vi "Sweep Control.vi"() -> ()   [LabVIEW 2019, in "SweepControl.lvclass"]
doc: "- Priority 0 is the fastest loop\n- You can put multiple scan names in one priority.\n- OFF has to be the last priority\n- Choose an Experiment (Lockin_Sweep, IV, etc) to run at each Scan Setting\n- Open the Exeriment subVIs to choose settings"
uses:
  SweepControl.lvclass
  Typedefs/Enum - Priority.ctl
  Typedefs/Enum - Action.ctl
  Typedefs/Cluster - ScanControl.ctl
  Typedefs/ScanControl.ctl
  Typedefs/Cluster - ScanParamters.ctl
  Typedefs/ScanParamters.ctl
  Typedefs/Enum - Experiments.ctl
  Typedefs/Sweep Control JSON--Cluster.ctl
  Control Experiment/Control Experiment.lvclass
  Typedefs/Enum - PostAction.ctl
  Typedefs/PostAction.ctl
  Typedefs/Enum - PostAction - 2.ctl
  Typedefs/Cluster - Sweep Control.ctl
panel:
  out "Repeat #":i32
  in  "Repeat Experiment":i32=100 caption="Repeat Experiment (at each parameter)" min=1
  in  "Stop":bool
  in  "Scan parameters 2":T1[](array[typedef]) {"Rate" format="%.2f"; "Step" format="%#_6p"; "End" format="%#_6p"; "Start" format="%#_6p"}
  in  "OK":bool
  in  "Experiment Description":string="T = 20 K\nRainbow 2 power = 250 uW before int\n50 second time delay scan [-0.5 ps, 0.5 ps]\n15 averages per Vgr value\n\ntop nanojunction Vsd = -0.7 V\nbottom nanojunction Vsd = -0.5 V\nVgr = 0 V\n\nSweep Vnw from 0 V to -1 V, -100 mV step\n\n"
  in  "Experiment subVI":T5=enum."THz_DelayLine"
  in  "Post action (indexing priority)":T6=[enum."Do Nothing", enum."Do Nothing", enum."Do Nothing", enum."Do Nothing"]
  in  "Experiment Folder (## - Description)":string="35 - sweep Vnw bottom 100 repeats "
  in  "Scan parameters":T8=[{"Start"=-0.5, "End"=-1.5, "Step"=0.1, "Rate"=0.0, "wait (ms/mK)"=2000, "Address"="Dev2/ao0", "channel"=5}, {"Start"=0.0, "End"=-1.0, "Step"=0.1, "Rate"=0.0, "wait (ms/mK)"=2000, "Address"="Dev2/ao0", "channel"=7}, {"Start"=0.2, "End"=0.3, "Step"=0.025, "Rate"=2.0, "wait (ms/mK)"=250, "Address"="Dev2/ao0", "channel"=3}, {"Start"=0.0, "End"=10000.0, "Step"=5000.0, "Rate"=0.0, "wait (ms/mK)"=0, "Address"="Dev2/ao0", "channel"=3}] {"Rate" format="%.2f"; "Step" format="%#_6p"; "End" format="%#_6p"; "Start" format="%#_6p"}
  in  "Scan control":T10=[{"Priority"=enum."Priority 0", "Scan name"=enum."Lockin Bias"}, {"Priority"=enum."Priority 0", "Scan name"=enum."Lockin Bias"}, {"Priority"=enum."Priority 2", "Scan name"=enum."OFF"}, {"Priority"=enum."Priority 3", "Scan name"=enum."OFF"}]
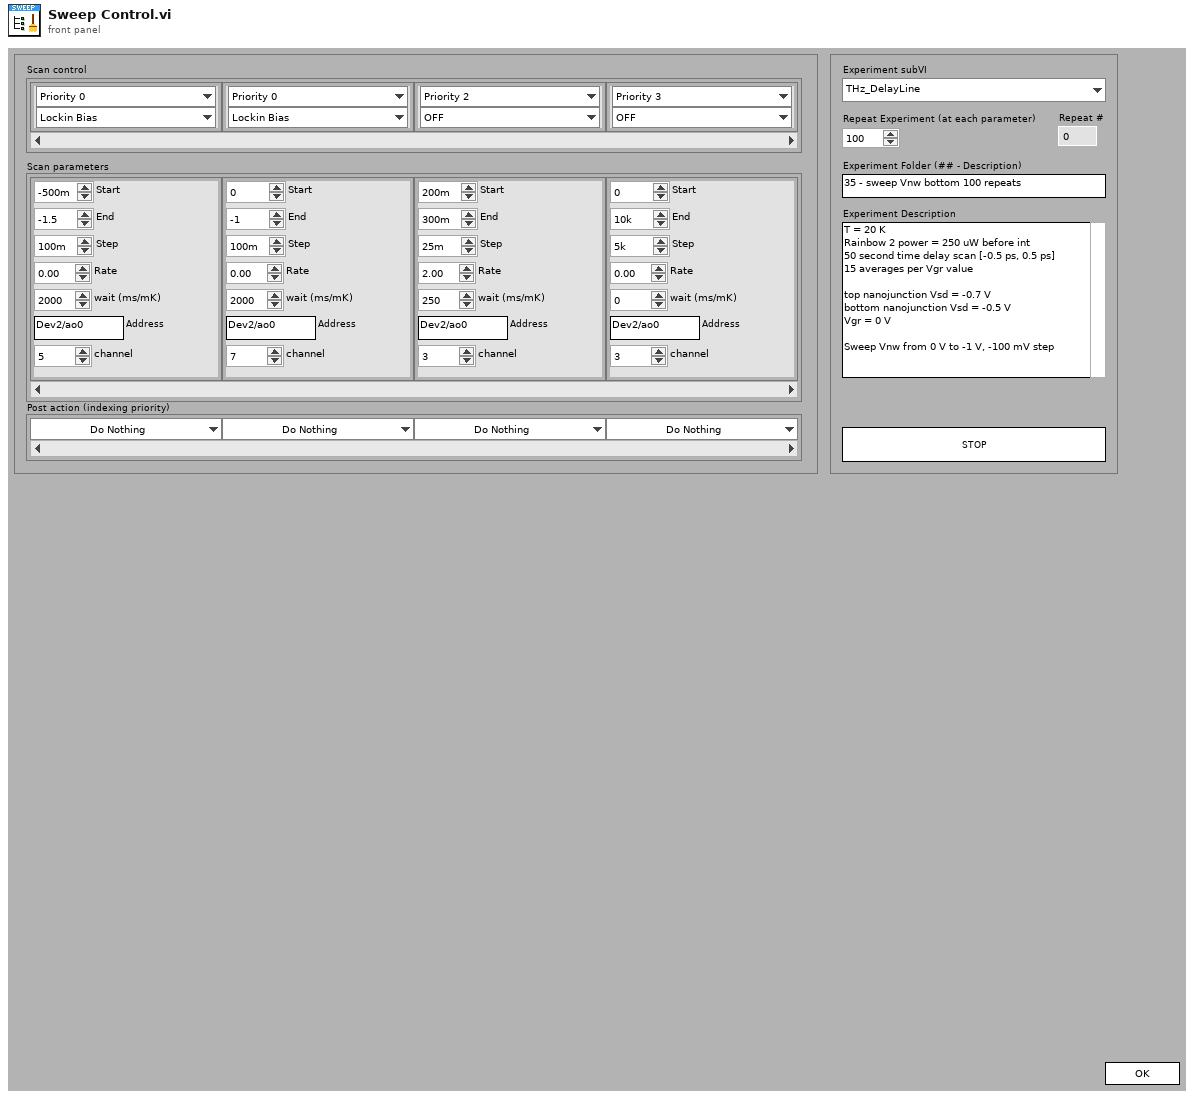
[diagram p1: front panel]
types:
  T1 = typedef "SweepControl.lvclass/Cluster - Sweep Control.ctl" = cluster{"Start":dbl, "End":dbl, "Step":dbl, "Rate":dbl, "wait (ms/mK)":u32, "Address":string, "Priority":T2, "Scan name":T3, "Post Actions":T4[], "channel":i32}
  T2 = typedef "SweepControl.lvclass/Enum - Priority.ctl" = enum16{"Priority 0", "Priority 1", "Priority 2", "Priority 3", "Priority 4", "Priority 5"}
  T3 = typedef "SweepControl.lvclass/Enum - Action.ctl" = enum16{"OFF", "time", "Lockin Amplitude", "Lockin Frequency", "Lockin Bias", "Delay", "Strain", "DAQ Bias", "Magnet Field", "Temperature", "MW f1", "MW f2", "MW Amplitude1", "MW Amplitude2"}
  T4 = typedef "SweepControl.lvclass/Enum - PostAction - 2.ctl" = enum16{"Do Nothing", "Wait (time)", "Wait (Temperature)", "Wait (<T ; B sweep)", "Wait (Magnet)"}
  T5 = typedef "SweepControl.lvclass/Enum - Experiments.ctl" = enum16{"IV", "IV_Fast", "IV_Sweep", "THz_DelayLine", "Lockin_Vsg", "Lockin_Sweep", "Lockin_Time", "AI WFM time", "Lockin (experimental)"}
  T6 = typedef "SweepControl.lvclass/PostAction.ctl" = T7[]
  T7 = typedef "SweepControl.lvclass/Enum - PostAction.ctl" = enum16{"Do Nothing", "Wait (time)", "Wait (Temperature)", "Wait (<T ; B sweep)", "Wait (Magnet)"}
  T8 = typedef "SweepControl.lvclass/ScanParamters.ctl" = T9[]
  T9 = typedef "SweepControl.lvclass/Cluster - ScanParamters.ctl" = cluster{"Start":dbl, "End":dbl, "Step":dbl, "Rate":dbl, "wait (ms/mK)":u32, "Address":string, "channel":i32}
  T10 = typedef "SweepControl.lvclass/ScanControl.ctl" = T11[]
  T11 = typedef "SweepControl.lvclass/Cluster - ScanControl.ctl" = cluster{"Priority":T2, "Scan name":T3}
  T12 = enum32{"Invalid", "Standard", "Closed", "Hidden", "Minimized", "Maximized"}
  T13 = enum32{"invalid app kind", "Development System", "Run Time System", "Student Edition", "Embedded LabVIEW", "Evaluation", "Custom"}
  T14 = cluster{"Core":cluster{"Current VI Reference":refnum<vi>, "Close Panel on Exit?":bool}, "SweepControl":refnum<class "SweepControl.lvclass">}
  T15 = cluster{"Current VI Reference":refnum<vi>, "Close Panel on Exit?":bool}
  T16 = typedef "SweepControl.lvclass/Sweep Control JSON--Cluster.ctl" = cluster{"Experiment":T5, "Repeat Experiment":i32, "Scan control":T10, "Scan parameters":T8}
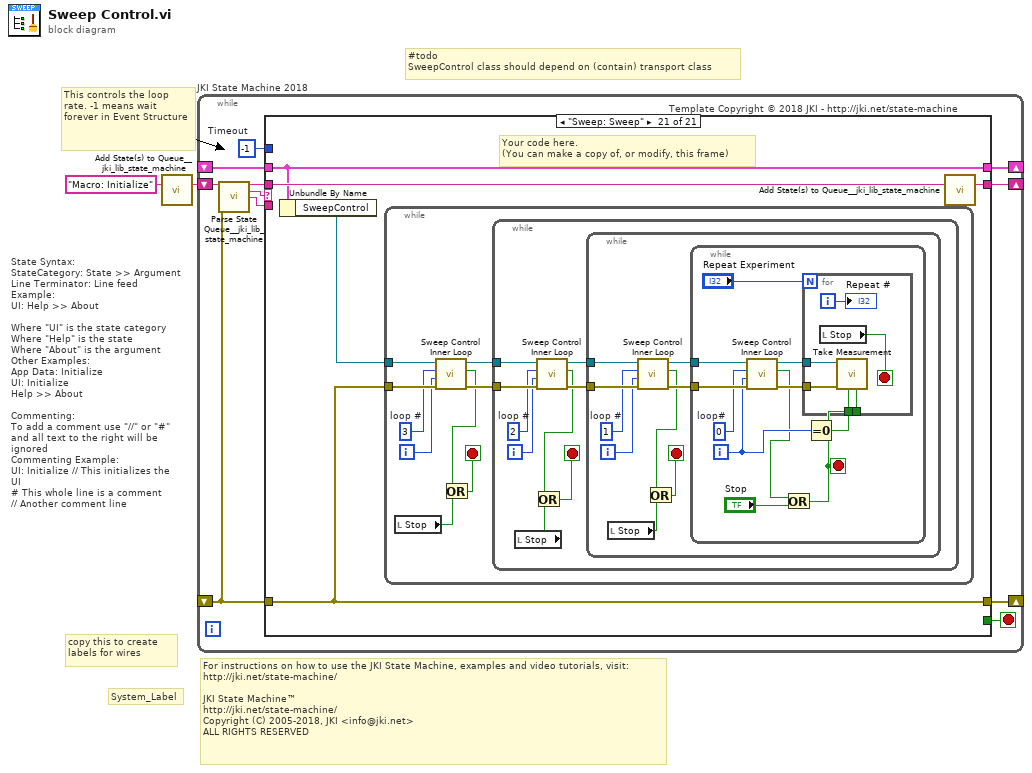
[diagram p0: block diagram]
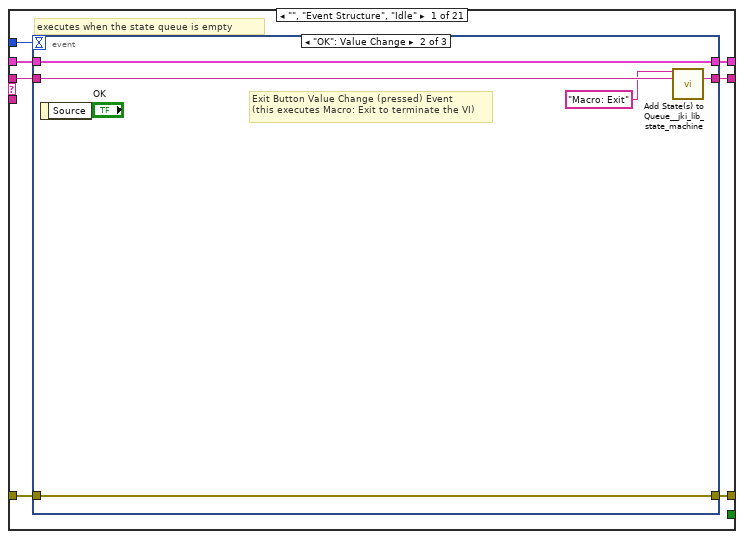
[diagram p2: hidden frame]
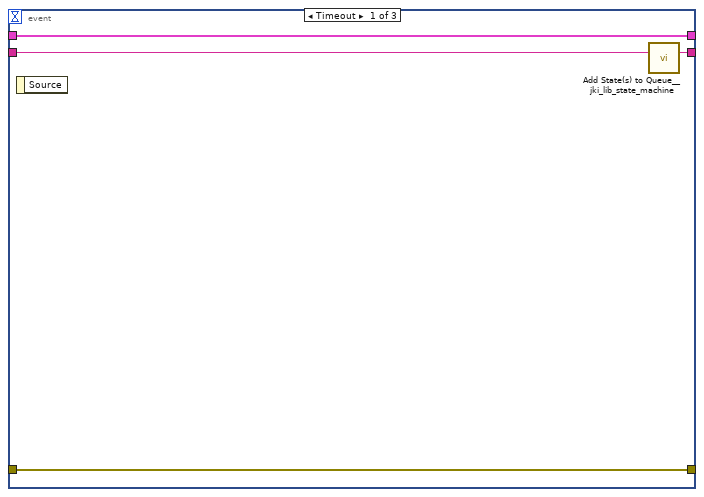
[diagram p3: hidden frame]
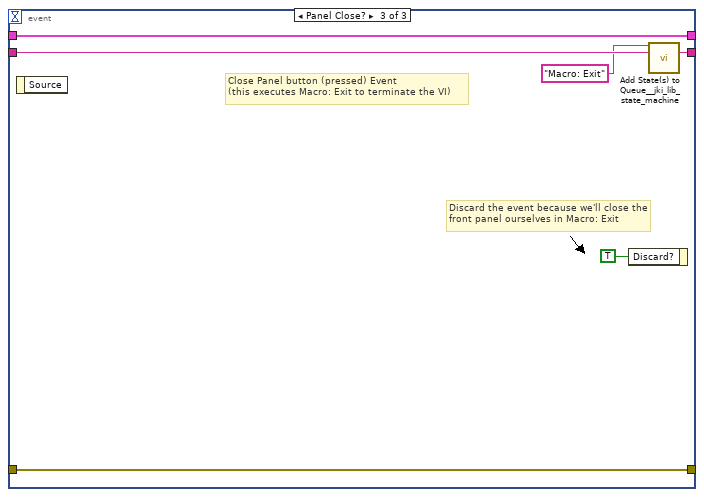
[diagram p4: hidden frame]
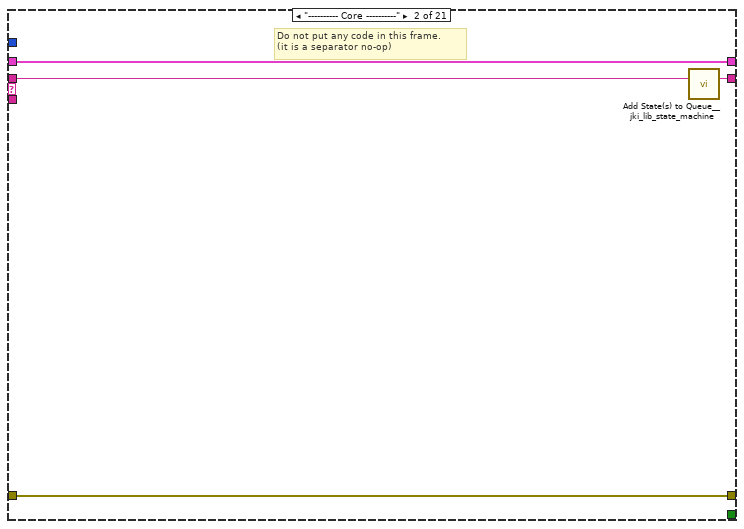
[diagram p5: hidden frame]
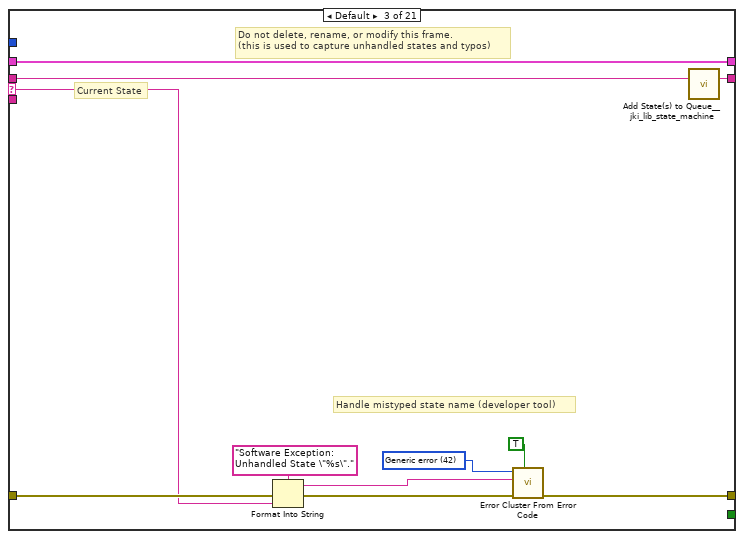
[diagram p6: hidden frame]
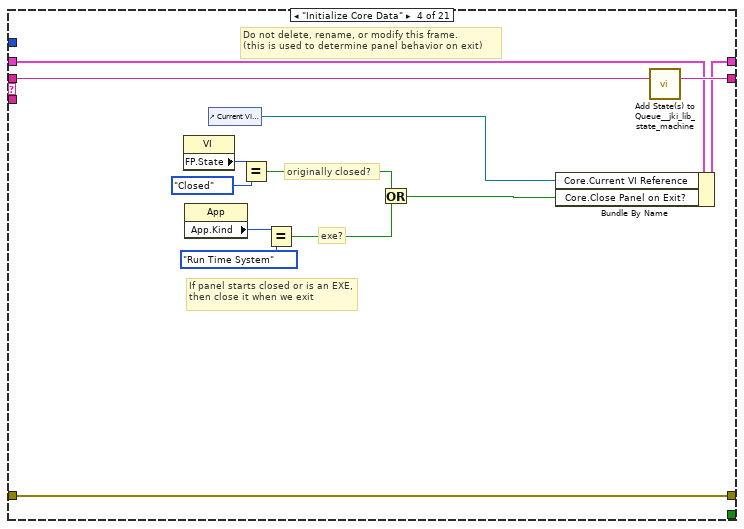
[diagram p7: hidden frame]
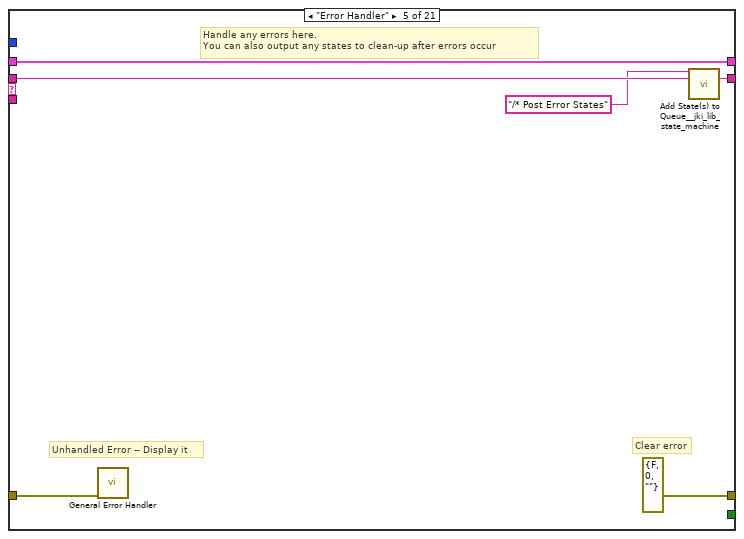
[diagram p8: hidden frame]
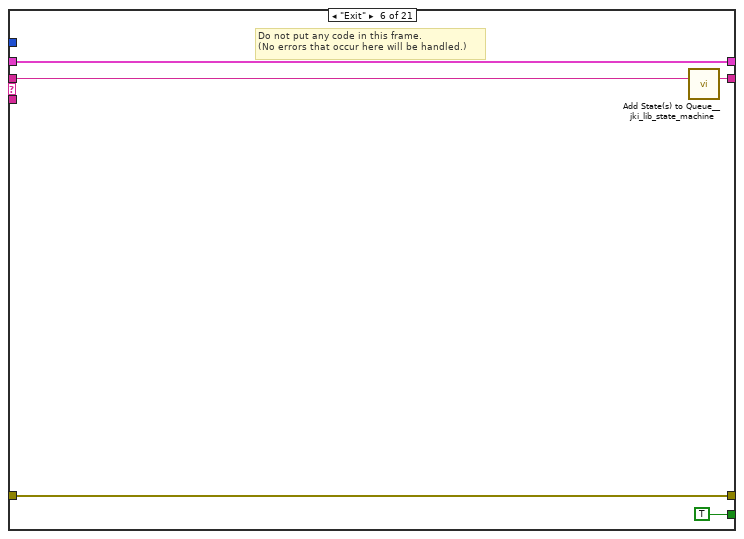
[diagram p9: hidden frame]
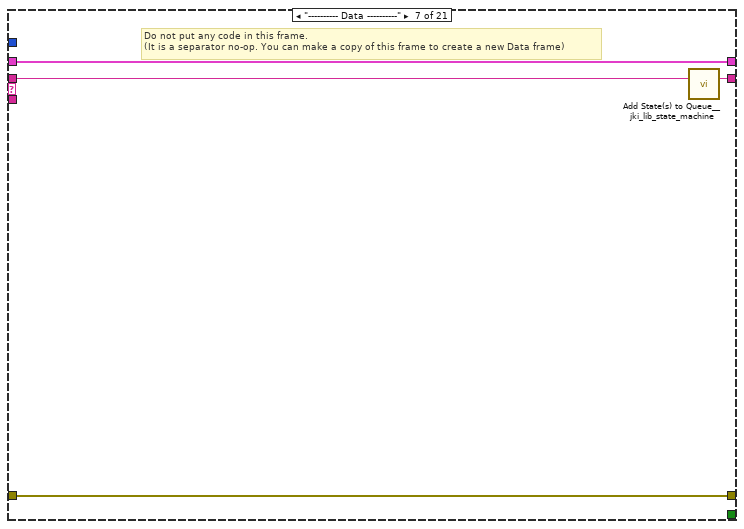
[diagram p10: hidden frame]
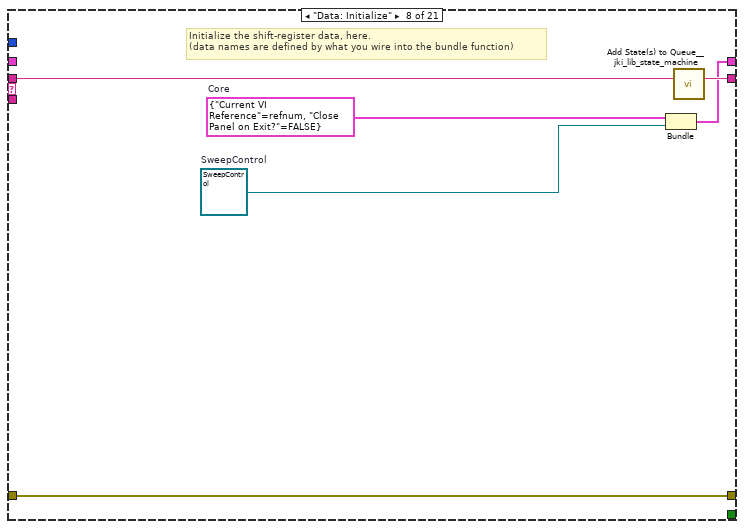
[diagram p11: hidden frame]
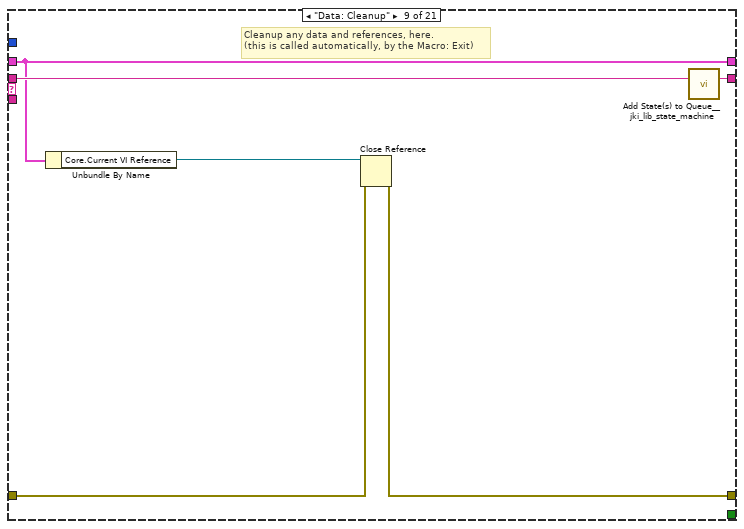
[diagram p12: hidden frame]
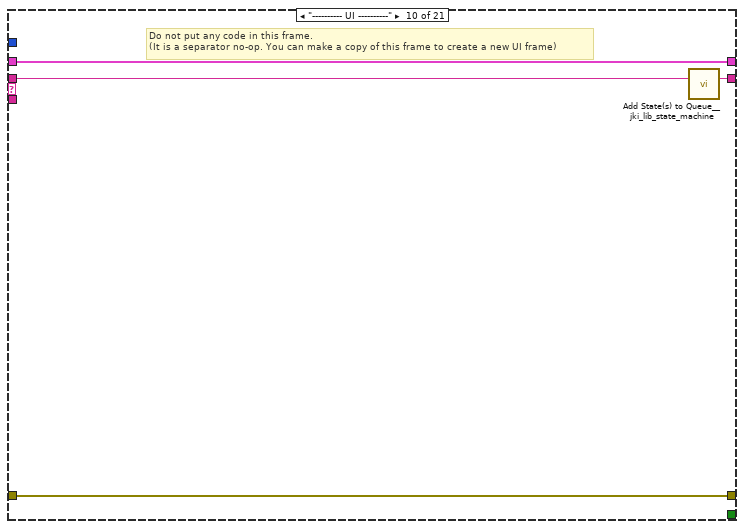
[diagram p13: hidden frame]
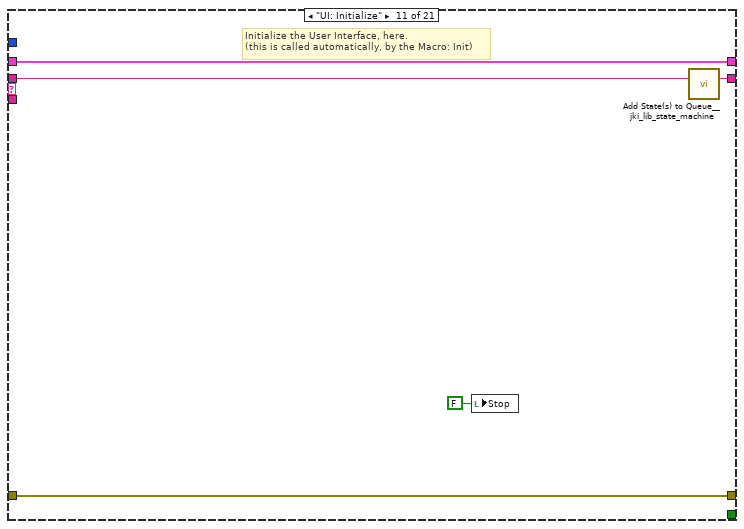
[diagram p14: hidden frame]
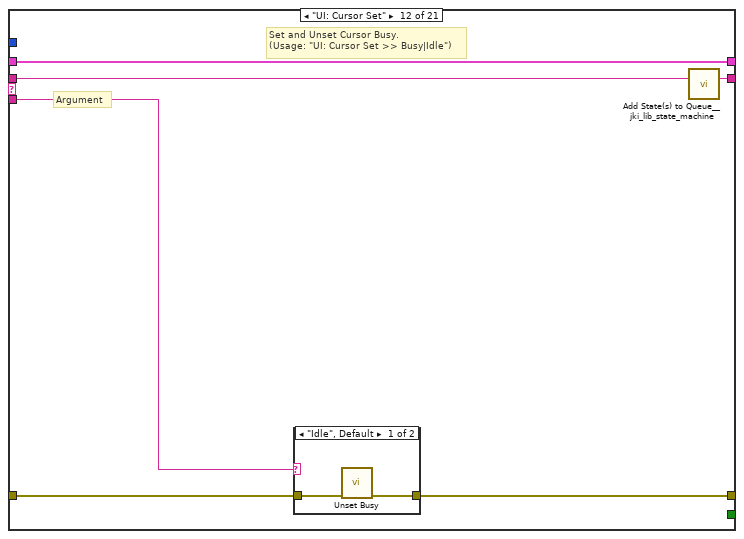
[diagram p15: hidden frame]
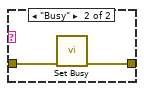
[diagram p16: hidden frame]
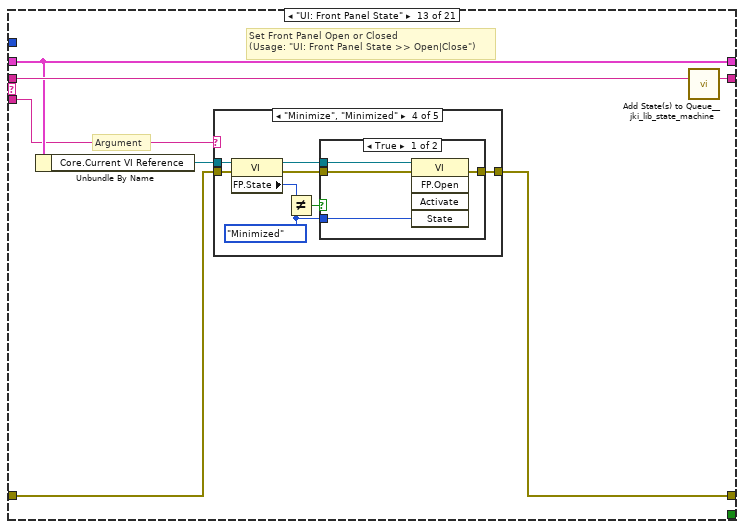
[diagram p17: hidden frame]
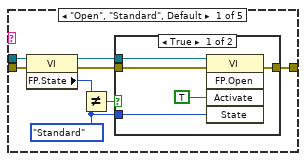
[diagram p18: hidden frame]
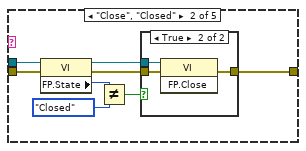
[diagram p20: hidden frame]
diagram:
  # "For instructions on how to use the JKI State Machine, examples and video tutorials, visit:\nhttp://jki.net/state-machine/\n\nJKI State Machine™\nhttp://jki.net/state-machine/\nCopyright (C) 2005-2018, JKI <info@jki.net>\nALL RIGHTS RESERVED"
  # "State Syntax:\nStateCategory: State >> Argument\nLine Terminator: Line feed\nExample:\nUI: Help >> About\n\nWhere \"UI\" is the state category\nWhere \"Help\" is the state\nWhere \"About\" is the argument\nOther Examples:\nApp Data: Initialize\nUI: Initialize\nHelp >> About\n\nCommenting:\nTo add a comment use \"//\" or \"#\" and all text to the right will be ignored\nCommenting Example:\nUI: Initialize // This initializes the UI\n# This whole line is a comment\n// Another comment line"
  # "copy this to create labels for wires"
  # "This controls the loop rate. -1 means wait forever in Event Structure"
  # "System_Label"
  # "#todo\nSweepControl class should depend on (contain) transport class"
  n1 = call <vilib>:"Add State(s) to Queue__jki_lib_state_machine.vi"("State(s) in (\"\")"="Macro: Initialize") -> ("States Out"=w2:string)  [unwired: 14 in]
  n2 = while "JKI State Machine 2018" {
    shift-right: [w6] -> _
    shift-left: _ -> [w5]
    shift-right: [w9] -> _
    shift-left: _ -> [w3]
    shift-right: [w8] -> _
    shift-left: w2 -> [w10]
    stop <- w7 stop-if-true
    w4 = -1  # Timeout
    # "Template Copyright © 2018 JKI - http://jki.net/state-machine"
    n3 = call <vilib>:"Parse State Queue__jki_lib_state_machine.vi"("State Queue"=w10, "Error In (no error)"=w3) -> ("Remaining States"=w12:string, "Current State"=w13:string, "Arguments"=w11:string)  [unwired: 11 in]
    n4 = case shown="\"Sweep: Sweep\"" w13 {
      selector: w13 -> [_ _ w40 _ _ _ _ _ _ _ _ _ _ _ _ _ _ _ _ _ _]
      tunnel: w12 -> [w20 w39 w44 w63 w69 w74 w78 w84 w90 w94 w99 w105 w116 w185 w190 w195 w205 w209 w234 w247 w251]
      tunnel: w11 -> [_ _ _ _ _ _ _ _ _ _ _ w100 w110 _ _ _ _ _ _ _ _]
      tunnel: w5 -> [w18 w36 w42 w56 w66 w72 w75 _ w85 w91 w97 w103 w112 w182 w187 w192 w202 w206 w228 w245 w250]
      tunnel: [w17 w37 w46 w60 errorcluster {"status"=FALSE, "code"=0, "source"=""} ("error out") w71 w76 w81 w86 w92 w96 w101 w113 w183 w188 w193 w203 w207 w226 w243 w249] -> w9
      tunnel: w3 -> [w16 w37 w45 w60 w65 w71 w76 w81 w87 w92 w96 w102 w114 w183 w188 w193 w203 w207 w222 w235 w249]
      tunnel: [w19 w38 w43 w62 w68 w73 w77 w83 w89 w93 w98 w104 w115 w184 w189 w194 w204 w208 w233 w246 w252] -> w8
      tunnel: [_ _ _ _ _ TRUE _ _ _ _ _ _ _ _ _ _ _ _ _ _ _] -> w7
      tunnel: [w15 w36 w42 w61 w66 w72 w75 w82 w85 w91 w97 w103 w112 w182 w187 w192 w202 w206 w227 w245 w250] -> w6
      tunnel: w4 -> [w14 _ _ _ _ _ _ _ _ _ _ _ _ _ _ _ _ _ _ _ _]
      frame "", "Event Structure", "Idle" {
        # "executes when the state queue is empty"
        n5 = event shown="[1] \"OK\": Value Change" {
          selector: _ -> [_ _ _]
          dyn-events: _ -> [_ _ _]
          timeout: w14 -> [_ _ _]
          tunnel: w20 -> [w24 w29 w35]
          tunnel: [w23 w28 w34] -> w19
          tunnel: w18 -> [w21 w26 w32]
          tunnel: [w22 w27 w33] -> w17
          tunnel: w16 -> [w22 w27 w33]
          tunnel: [w21 w26 w32] -> w15
          event Timeout {
            n6 = event-data() -> ()  [unwired: 1 in, 1 out]
            n7 = call <vilib>:"Add State(s) to Queue__jki_lib_state_machine.vi"("State(s) in (\"\")"=w24) -> ("States Out"=w23:string)  [unwired: 14 in]
          }
          event "OK": Value Change {
            # "Exit Button Value Change (pressed) Event\n(this executes Macro: Exit to terminate the VI)"
            n8 = event-data() -> ()  [unwired: 1 in, 1 out]
            n9 = call <vilib>:"Add State(s) to Queue__jki_lib_state_machine.vi"("State(s) in Front (\"\")"="Macro: Exit", "State(s) in (\"\")"=w29) -> ("States Out"=w28:string)  [unwired: 13 in]
          }
          event Panel Close? {
            # "Discard the event because we'll close the front panel ourselves in Macro: Exit"
            # "Close Panel button (pressed) Event\n(this executes Macro: Exit to terminate the VI)"
            n10 = event-data() -> ()  [unwired: 1 in, 1 out]
            n11 = event-data("Discard?"=TRUE) -> ()  [unwired: 1 in, 1 out]
            n12 = call <vilib>:"Add State(s) to Queue__jki_lib_state_machine.vi"("State(s) in Front (\"\")"="Macro: Exit", "State(s) in (\"\")"=w35) -> ("States Out"=w34:string)  [unwired: 13 in]
          }
        }
      }
      frame "---------- Core ----------" {
        # "Do not put any code in this frame.\n(it is a separator no-op)"
        n13 = call <vilib>:"Add State(s) to Queue__jki_lib_state_machine.vi"("State(s) in (\"\")"=w39) -> ("States Out"=w38:string)  [unwired: 14 in]
      }
      frame Default {
        w49 = 42 items=["No error", "Argument error", "Memory is full", "Out of zone", "End of file", "File already open", "Generic file I/O error", "File not found", "File permission error", "Disk is full", "Duplicate path", "Too many files open", "System feature not enabled", "Resource file not found", "Cannot add resource", "Resource not found", "Image not found", "Image memory error", "Pen does not exist", "Config type invalid", "Config token not found", "Config parse error", "Config memory error", "Bad external code format", "Bad external code offset", "External code not present", "Null window", "Destroy window error", "Null menu", "Print aborted", "Bad print record", "Print driver error", "Windows error during printing", "Memory error during printing", "Print dialog error", "Generic print error", "Invalid device refnum", "Device not found", "Device parameter error", "Device unit error", "Cannot open device", "Device call aborted", "Generic error", "Cancelled by user", "Object ID too low", "Object ID too high", "Object not in heap", "Unknown heap", "Unknown object (invalid DefProc)", "Unknown object (DefProc not in table)", "Message out of range", "Invalid (null) method", "Unknown message", "Manager call not supported", "Bad address", "Network operation in progress", "Network operation timed out", "Connection is busy", "Network attribute not supported", "Network error", "Address in use", "System out of memory", "Connection aborted", "Connection refused", "Not connected", "Already connected", "Connection closed", "Initialization error (interapplication manager)", "Bad occurrence", "Wait on unbound occurrence handler", "Occurrence queue overflow", "Datalog type conflict", "Unused", "Unrecognized type (interapplication manager)", "Memory corrupt", "Failed to make temporary DLL", "Old CIN version", "Drag socket not found", "Failed to load drop-object", "Failed to register OLE object", "Failed to release OLE object", "Format specifier type mismatch", "Unknown format specifier", "Too few format specifiers", "Too many format specifiers", "Scan failed", "Newer CIN version", "Error converting to variant", "Runtime menu error", "Password tampered", "Variant attribute not found", "Incompatible variant data type", "Event data is not available", "Event Store is not present", "Occurrence is not found", "Event Queue is not created", "Event info is not available", "Refnum passed is NULL", "Error retrieving Class GUID", "Error retrieving CoClass GUID", "Error retrieving TypeLib GUID.", "Bad built application magic bytes.", "Specific driver is different from the specific driver associated with the Logical Name.", "There is no session opened to the class driver.", "Max Error", "MAX - Error with config objects", "MAX - Error loading configuration", "MAX - Group not supported"]
        # "Current State"
        # "Do not delete, rename, or modify this frame.\n(this is used to capture unhandled states and typos)"
        # "Handle mistyped state name (developer tool)"
        n14 = Format Into String(format string="Software Exception: Unhandled State \"%s\"." ("message"), error in=w45, w40) -> (resulting string=w48:string, error out=w47:errorcluster)  [unwired: 1 in]
        n15 = call <vilib>:"Error Cluster From Error Code.vi"("show call chain? (False)"=TRUE, "error in (no error)"=w47, "error message (\"\")"=w48, "error code (0)"=w49) -> ("error out"=w46:errorcluster)  [unwired: 5 in]
        n16 = call <vilib>:"Add State(s) to Queue__jki_lib_state_machine.vi"("State(s) in (\"\")"=w44) -> ("States Out"=w43:string)  [unwired: 14 in]
      }
      frame "Initialize Core Data" {
        # "Do not delete, rename, or modify this frame.\n(this is used to determine panel behavior on exit)"
        # "originally closed?"
        # "exe?"
        # "If panel starts closed or is an EXE, then close it when we exit"
        n17 = property class="VI"() -> ("FP.State"=w53:T12)  [unwired: 2 in, 2 out]
        n18 = property class="App"() -> ("App.Kind"=w59:T13)  [unwired: 2 in, 2 out]
        n19 = control-ref of="Current VI Reference"() -> (w54:refnum<vi>)
        n20 = Equal?(x=w53, y=T12."Closed" ("Front Panel Window:State")) -> (x = y?=w51:bool)
        n21 = Equal?(x=w59, y=T13."Run Time System" ("Application:Kind")) -> (x = y?=w57:bool)
        n22 = Or(x=w51, y=w57) -> (x .or. y?=w55:bool)
        n23 = Bundle By Name(cluster=w56, "Core.Current VI Reference"=w54, "Core.Close Panel on Exit?"=w55) -> (w61:T14)
        n24 = call <vilib>:"Add State(s) to Queue__jki_lib_state_machine.vi"("State(s) in (\"\")"=w63) -> ("States Out"=w62:string)  [unwired: 14 in]
      }
      frame "Error Handler" {
        # "Unhandled Error -- Display it"
        # "Handle any errors here.\nYou can also output any states to clean-up after errors occur"
        # "Clear error"
        n25 = call <vilib>:"General Error Handler.vi"("error in (no error)"=w65) -> ()  [unwired: 10 in, 5 out]
        n26 = call <vilib>:"Add State(s) to Queue__jki_lib_state_machine.vi"("State(s) in Front (\"\")"="/* Post Error States", "State(s) in (\"\")"=w69) -> ("States Out"=w68:string)  [unwired: 13 in]
      }
      frame "Exit" {
        # "Do not put any code in this frame.\n(No errors that occur here will be handled.)"
        n27 = call <vilib>:"Add State(s) to Queue__jki_lib_state_machine.vi"("State(s) in (\"\")"=w74) -> ("States Out"=w73:string)  [unwired: 14 in]
      }
      frame "---------- Data ----------" {
        # "Do not put any code in this frame.\n(It is a separator no-op. You can make a copy of this frame to create a new Data frame)"
        n28 = call <vilib>:"Add State(s) to Queue__jki_lib_state_machine.vi"("State(s) in (\"\")"=w78) -> ("States Out"=w77:string)  [unwired: 14 in]
      }
      frame "Data: Initialize" {
        w79 = refnum<class "SweepControl.lvclass"> refnum  # SweepControl
        w80 = T15 {"Current VI Reference"=refnum, "Close Panel on Exit?"=FALSE}  # Core
        # "Initialize the shift-register data, here.\n(data names are defined by what you wire into the bundle function)"
        n29 = Bundle("Core"=w80, "SweepControl"=w79) -> (w82:T14)  [unwired: 1 in]
        n30 = call <vilib>:"Add State(s) to Queue__jki_lib_state_machine.vi"("State(s) in (\"\")"=w84) -> ("States Out"=w83:string)  [unwired: 14 in]
      }
      frame "Data: Cleanup" {
        # "Cleanup any data and references, here.\n(this is called automatically, by the Macro: Exit)"
        n31 = Unbundle By Name(w85) -> ("Core.Current VI Reference"=w88:refnum<vi>)
        n32 = Close Reference(reference=w88, error in (no error)=w87) -> (error out=w86:errorcluster)
        n33 = call <vilib>:"Add State(s) to Queue__jki_lib_state_machine.vi"("State(s) in (\"\")"=w90) -> ("States Out"=w89:string)  [unwired: 14 in]
      }
      frame "---------- UI ----------" {
        # "Do not put any code in this frame.\n(It is a separator no-op. You can make a copy of this frame to create a new UI frame)"
        n34 = call <vilib>:"Add State(s) to Queue__jki_lib_state_machine.vi"("State(s) in (\"\")"=w94) -> ("States Out"=w93:string)  [unwired: 14 in]
      }
      frame "UI: Initialize" {
        # "Initialize the User Interface, here.\n(this is called automatically, by the Macro: Init)"
        n35 = local write "Stop"(FALSE ("Stop")) -> ()
        n36 = call <vilib>:"Add State(s) to Queue__jki_lib_state_machine.vi"("State(s) in (\"\")"=w99) -> ("States Out"=w98:string)  [unwired: 14 in]
      }
      frame "UI: Cursor Set" {
        # "Argument"
        # "Set and Unset Cursor Busy.\n(Usage: \"UI: Cursor Set >> Busy|Idle\")"
        n37 = case shown="\"Idle\", Default" w100 {
          tunnel: w102 -> [w107 w109]
          tunnel: [w106 w108] -> w101
          frame "Idle", Default {
            n38 = call <vilib>:"Unset Busy.vi"("error in (no error)"=w107) -> ("error out"=w106:errorcluster)  [unwired: 10 in]
          }
          frame "Busy" {
            n39 = call <vilib>:"Set Busy.vi"("error in (no error)"=w109) -> ("error out"=w108:errorcluster)  [unwired: 9 in, 1 out]
          }
        }
        n40 = call <vilib>:"Add State(s) to Queue__jki_lib_state_machine.vi"("State(s) in (\"\")"=w105) -> ("States Out"=w104:string)  [unwired: 14 in]
      }
      frame "UI: Front Panel State" {
        # "Argument"
        # "Set Front Panel Open or Closed\n(Usage: \"UI: Front Panel State >> Open|Close\")"
        n41 = Unbundle By Name(w112) -> ("Core.Current VI Reference"=w111:refnum<vi>)
        n42 = case shown="\"Minimize\", \"Minimized\"" w110 {
          tunnel: w114 -> [w122 w137 w148 w161 w174]
          tunnel: [w124 w138 w150 w163 w176] -> w113
          tunnel: w111 -> [w123 w135 w149 w162 w175]
          frame "Open", "Standard", Default {
            w117 = T12."Standard" ("State")
            n43 = property class="VI"(reference=w123, error in=w122) -> (reference out=w120:refnum<vi>, error out=w121:errorcluster, "FP.State"=w119:T12)
            n44 = Not Equal?(x=w119, y=w117) -> (x != y?=w118:bool)
            n45 = case shown="True" w118 {
              tunnel: [w128 w130] -> w124
              tunnel: w121 -> [w127 w130]
              tunnel: w120 -> [w126 _]
              tunnel: w117 -> [w125 _]
              frame True {
                n46 = invoke class="VI" method="FP.Open"(reference=w126, error in=w127, "Activate"=TRUE, "State"=w125) -> (error out=w128:errorcluster)  [unwired: 1 in, 4 out]
              }
              frame False {
              }
            }
          }
          frame "Close", "Closed" {
            n47 = property class="VI"(reference=w135, error in=w137) -> (reference out=w134:refnum<vi>, error out=w136:errorcluster, "FP.State"=w132:T12)
            n48 = Not Equal?(x=w132, y=T12."Closed" ("Front Panel Window:State")) -> (x != y?=w131:bool)
            n49 = case shown="True" w131 {
              tunnel: [w139 w142] -> w138
              tunnel: w136 -> [w139 w141]
              tunnel: w134 -> [_ w140]
              frame False {
              }
              frame True {
                n50 = invoke class="VI" method="FP.Close"(reference=w140, error in=w141) -> (error out=w142:errorcluster)  [unwired: 1 in, 2 out]
              }
            }
          }
          frame "Hidden", "Hide" {
            w143 = T12."Hidden" ("State")
            n51 = property class="VI"(reference=w149, error in=w148) -> (reference out=w146:refnum<vi>, error out=w147:errorcluster, "FP.State"=w145:T12)
            n52 = Not Equal?(x=w145, y=w143) -> (x != y?=w144:bool)
            n53 = case shown="True" w144 {
              tunnel: [w154 w155] -> w150
              tunnel: w147 -> [w153 w155]
              tunnel: w146 -> [w152 _]
              tunnel: w143 -> [w151 _]
              frame True {
                n54 = invoke class="VI" method="FP.Open"(reference=w152, error in=w153, "State"=w151) -> (error out=w154:errorcluster)  [unwired: 2 in, 4 out]
              }
              frame False {
              }
            }
          }
          frame "Minimize", "Minimized" {
            w156 = T12."Minimized" ("State")
            n55 = property class="VI"(reference=w162, error in=w161) -> (reference out=w159:refnum<vi>, error out=w160:errorcluster, "FP.State"=w158:T12)
            n56 = Not Equal?(x=w158, y=w156) -> (x != y?=w157:bool)
            n57 = case shown="True" w157 {
              tunnel: [w167 w168] -> w163
              tunnel: w160 -> [w166 w168]
              tunnel: w159 -> [w165 _]
              tunnel: w156 -> [w164 _]
              frame True {
                n58 = invoke class="VI" method="FP.Open"(reference=w165, error in=w166, "State"=w164) -> (error out=w167:errorcluster)  [unwired: 2 in, 4 out]
              }
              frame False {
              }
            }
          }
          frame "Maximize", "Maximized" {
            w169 = T12."Maximized" ("State")
            n59 = property class="VI"(reference=w175, error in=w174) -> (reference out=w172:refnum<vi>, error out=w173:errorcluster, "FP.State"=w171:T12)
            n60 = Not Equal?(x=w171, y=w169) -> (x != y?=w170:bool)
            n61 = case shown="True" w170 {
              tunnel: [w180 w181] -> w176
              tunnel: w173 -> [w179 w181]
              tunnel: w172 -> [w178 _]
              tunnel: w169 -> [w177 _]
              frame True {
                n62 = invoke class="VI" method="FP.Open"(reference=w178, error in=w179, "State"=w177) -> (error out=w180:errorcluster)  [unwired: 2 in, 4 out]
              }
              frame False {
              }
            }
          }
        }
        n63 = call <vilib>:"Add State(s) to Queue__jki_lib_state_machine.vi"("State(s) in (\"\")"=w116) -> ("States Out"=w115:string)  [unwired: 14 in]
      }
      frame "---------- Macro ----------" {
        # "Do not put any code in this frame.\n(It is a separator no-op. You can make a copy of this frame to create a new Macro frame)"
        n64 = call <vilib>:"Add State(s) to Queue__jki_lib_state_machine.vi"("State(s) in (\"\")"=w185) -> ("States Out"=w184:string)  [unwired: 14 in]
      }
      frame "Macro: Initialize" {
        w186 = "Data: Initialize\nInitialize Core Data\nUI: Initialize\nUI: Front Panel State >> Open\nMacro: Sweep"  # Data: Initialize Initialize Core Data UI: Initialize UI: Front Panel State >> Open Macro: Sweep
        # "Initialization Macro\n(This is called once, when the VI starts)"
        n65 = call <vilib>:"Add State(s) to Queue__jki_lib_state_machine.vi"("State(s) in Front (\"\")"=w186, "State(s) in (\"\")"=w190) -> ("States Out"=w189:string)  [unwired: 13 in]
      }
      frame "Macro: Sweep" {
        # "Do not put any code in this frame.\n(It is a separator no-op. You can make a copy of this frame to create a new Macro frame)"
        n66 = call <vilib>:"Add State(s) to Queue__jki_lib_state_machine.vi"("State(s) in Front (\"\")"="Sweep: Initialize\nSweep: Write JSON File\nSweep: Sweep\nMacro: Exit", "State(s) in (\"\")"=w195) -> ("States Out"=w194:string)  [unwired: 13 in]
      }
      frame "Macro: Exit" {
        # "Exit Macro\n(This is called once, when the VI exits)"
        n67 = Unbundle By Name(w202) -> ("Core.Close Panel on Exit?"=w201:bool)
        n68 = Select(t="UI: Front Panel State >> Close", s=w201, f="") -> (s? t:f=w198:string)
        n69 = call <vilib>:"Add State(s) to Queue__jki_lib_state_machine.vi"("State(s) in (\"\")"=w198, "State(s) at Back (\"\")"="Data: Cleanup\nExit") -> ("States Out"=w196:string)  [unwired: 13 in]
        n70 = call <vilib>:"Add State(s) to Queue__jki_lib_state_machine.vi"("State(s) in Front (\"\")"=w196, "State(s) in (\"\")"=w205) -> ("States Out"=w204:string)  [unwired: 13 in]
      }
      frame "---------- Sweep ----------" {
        # "Template Separator\n(You can make a copy of, or modify, this frame)"
        n71 = call <vilib>:"Add State(s) to Queue__jki_lib_state_machine.vi"("State(s) in (\"\")"=w209) -> ("States Out"=w208:string)  [unwired: 14 in]
      }
      frame "Sweep: Initialize" {
        # "hidden: 1/7/2020"
        # "Your code here.\n(You can make a copy of, or modify, this frame)"
        n72 = Unbundle By Name(w228) -> ("SweepControl"=w225:refnum<class "SweepControl.lvclass">)
        n73 = call "Control Experiment FGV.vi"("Function"=enum16{"read", "write"}."read", "error in (no error)"=w222) -> ("error out"=w214:errorcluster, "Control Experiment.lvclass out"=w216:refnum<class "Control Experiment.lvclass">)  [unwired: 8 in]
        n74 = call "Write Experiment Description.vi"("error in (no error)"=w214, "Experiment Description"="Experiment Description", "Control Experiment in"=w216) -> ("error out"=w213:errorcluster, "Control Experiment out"=w212:refnum<class "Control Experiment.lvclass">)  [unwired: 7 in]
        n75 = call "Write Experiment Folder.vi"("error in (no error)"=w213, "Experiment Folder"="Experiment Folder (## - Description)", "Control Experiment in"=w212) -> ("error out"=w218:errorcluster, "Control Experiment out"=w219:refnum<class "Control Experiment.lvclass">)  [unwired: 7 in]
        n76 = call "Read Instruments.vi"("error in (no error)"=w218, "Control Experiment in"=w219) -> ("error out"=w217:errorcluster, "Control Experiment out"=w211:refnum<class "Control Experiment.lvclass">)  [unwired: 7 in, 1 out]
        n77 = Bundle By Name(cluster=w225, "Scan control"="Scan control", "Scan parameters"="Scan parameters", "Post action (indexing priority)"="Post action (indexing priority)", "Experiment"="Experiment subVI", "Control Experiment"=w211, "Scan parameters 2"="Scan parameters 2") -> (w224:refnum<class "SweepControl.lvclass">)
        n78 = call "Sort Scan Parameters.vi"("error in (no error)"=w217, "SweepControl"=w224) -> ("error out"=w226:errorcluster, "SweepControl"=w220:refnum<class "SweepControl.lvclass">)  [unwired: 6 in, 2 out]
        n79 = Bundle By Name(cluster=w228, "SweepControl"=w220) -> (w227:T14)
        n80 = call <vilib>:"Add State(s) to Queue__jki_lib_state_machine.vi"("State(s) in (\"\")"=w234) -> ("States Out"=w233:string)  [unwired: 14 in]
      }
      frame "Sweep: Write JSON File" {
        w244 = T16 {"Experiment"=enum."IV", "Repeat Experiment"=0, "Scan control"=[], "Scan parameters"=[]}  # SweepControl
        # "Write JSON File\n(Writes Sweep Control configuration to *.json file)"
        n81 = Unbundle By Name(w245) -> ("SweepControl"=w238:refnum<class "SweepControl.lvclass">)
        n82 = Unbundle By Name(w238) -> ("Control Experiment"=w237:refnum<class "Control Experiment.lvclass">)
        n83 = local read "Repeat Experiment"() -> (w236:i32)
        n84 = Unbundle By Name(w238) -> ("Scan control"=w242:T10, "Scan parameters"=w241:T8, "Experiment"=w240:T5)
        n85 = Bundle By Name(cluster=w244, "Scan control"=w242, "Scan parameters"=w241, "Experiment"=w240, "Repeat Experiment"=w236) -> (w239:T16)
        n86 = call "Save JSON File.vi"("error in (no error)"=w235, "Data"=w239, "Control Experiment in"=w237) -> ("error out"=w243:errorcluster)  [unwired: 8 in]
        n87 = call <vilib>:"Add State(s) to Queue__jki_lib_state_machine.vi"("State(s) in (\"\")"=w247) -> ("States Out"=w246:string)  [unwired: 14 in]
      }
      frame "Sweep: Sweep" {
        # "Your code here.\n(You can make a copy of, or modify, this frame)"
        n88 = Unbundle By Name(w250) -> ("SweepControl"=w248:refnum<class "SweepControl.lvclass">)
        n89 = while {
          tunnel: w249 -> [w259]
          tunnel: w248 -> [w261]
          i -> [w256]
          stop <- w253 stop-if-true
          w257 = 3  # loop #
          n90 = local read "Stop"() -> (w255:bool)
          n91 = call "Sweep Control Inner Loop.vi"("error in (no error)"=w259, "inner loop index"=w256, "loop #"=w257, "SweepControl in"=w261) -> ("error out"=w258:errorcluster, "Stop?"=w254:bool, "SweepControl out"=w260:refnum<class "SweepControl.lvclass">)  [unwired: 5 in]
          n92 = Or(x=w254, y=w255) -> (x .or. y?=w253:bool)
          n93 = while {
            tunnel: w258 -> [w269]
            tunnel: w260 -> [w270]
            i -> [w265]
            stop <- w262 stop-if-true
            w268 = 2  # loop #
            n94 = local read "Stop"() -> (w264:bool)
            n95 = call "Sweep Control Inner Loop.vi"("error in (no error)"=w269, "inner loop index"=w265, "loop #"=w268, "SweepControl in"=w270) -> ("error out"=w267:errorcluster, "Stop?"=w263:bool, "SweepControl out"=w266:refnum<class "SweepControl.lvclass">)  [unwired: 5 in]
            n96 = Or(x=w263, y=w264) -> (x .or. y?=w262:bool)
            n97 = while {
              tunnel: w267 -> [w279]
              tunnel: w266 -> [w278]
              i -> [w274]
              stop <- w271 stop-if-true
              w277 = 1  # loop #
              n98 = local read "Stop"() -> (w273:bool)
              n99 = call "Sweep Control Inner Loop.vi"("error in (no error)"=w279, "inner loop index"=w274, "loop #"=w277, "SweepControl in"=w278) -> ("error out"=w276:errorcluster, "Stop?"=w272:bool, "SweepControl out"=w275:refnum<class "SweepControl.lvclass">)  [unwired: 5 in]
              n100 = Or(x=w272, y=w273) -> (x .or. y?=w271:bool)
              n101 = while {
                tunnel: w276 -> [w290]
                tunnel: w275 -> [w286]
                i -> [w285]
                stop <- w281 stop-if-true
                w289 = 0  # loop#
                n102 = call "Sweep Control Inner Loop.vi"("error in (no error)"=w290, "inner loop index"=w285, "loop #"=w289, "SweepControl in"=w286) -> ("error out"=w288:errorcluster, "Stop?"=w283:bool, "SweepControl out"=w287:refnum<class "SweepControl.lvclass">)  [unwired: 5 in]
                n103 = Or(x=w283, y="Stop") -> (x .or. y?=w281:bool)
                n104 = Equal To 0?(x=w285) -> (x = 0?=w284:bool)
                n105 = for {
                  N: "Repeat Experiment" -> [_]
                  tunnel: w288 -> [w296]
                  tunnel: w287 -> [w295]
                  tunnel: w284 -> [w294]
                  tunnel: w281 -> [w292]
                  i -> [w293]
                  stop <- w291 stop-if-true
                  n106 = local read "Stop"() -> (w291:bool)
                  n107 = call "Take Measurement.vi"("stop?"=w292, "initialize?"=w294, "error in (no error)"=w296, "SweepControl in"=w295) -> ()  [unwired: 7 in, 1 out]
                  "Repeat #" <- w293
                }
              }
            }
          }
        }
        n108 = call <vilib>:"Add State(s) to Queue__jki_lib_state_machine.vi"("State(s) in (\"\")"=w251) -> ("States Out"=w252:string)  [unwired: 14 in]
      }
    }
  }
